vi "Assert Count.vi"(5 "Expected":i32, 7 "Message (\"\")":string, 8 "error in (no error)":errorcluster, 10 "Haystack":variant) -> (0 "error out":errorcluster)   [LabVIEW 2017, in "Transparent Assertions.lvlib" / "Assertions.lvlib"]
doc: "Asserts that the number of elements in an array, set, or map matches the expected count. Returns an error if the assertion fails, and optionally appends a custom message to the error."
uses:
  Assertions.lvlib
  Constraints/Count/Count.lvclass
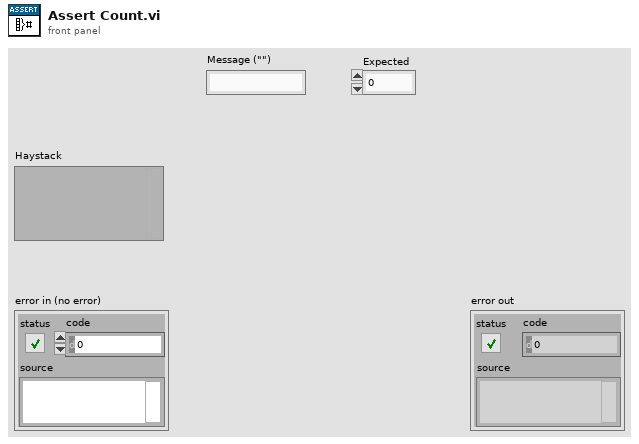
[diagram p1: front panel]
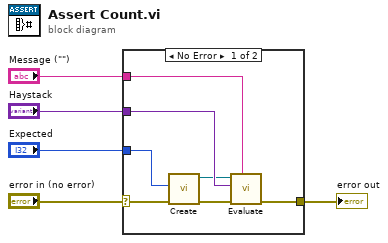
[diagram p0: block diagram]
diagram:
  n1 = case shown="No Error" "error in (no error)" {
    selector: "error in (no error)" -> [w6 w13]
    tunnel: [w12 w13] -> w5
    tunnel: "Haystack" -> [w11 _]
    tunnel: "Message (\"\")" -> [w10 _]
    tunnel: "Expected" -> [w9 _]
    frame No Error {
      n2 = call "Create.vi"("error in (no error)"=w6, "Expected"=w9) -> ("error out"=w8:errorcluster, "Count"=w7:refnum<class "Count.lvclass">)  [unwired: 8 in]
      n3 = call-dynamic "Evaluate.vi"("Message (\"\")"=w10, "error in (no error)"=w8, "Actual"=w11, "Constraint in"=w7) -> ("error out"=w12:errorcluster)  [unwired: 6 in, 1 out]
    }
    frame Error {
    }
  }
  "error out" <- w5
